vi "test SSL Client Read Before Write.vi"(8 "error in (no error)":errorcluster, 11 "TestCase in":refnum<class "test SSL Client.lvclass">) -> (0 "error out":errorcluster, 3 "TestCase out":refnum<class "test SSL Client.lvclass">)   [LabVIEW 2013, in "test SSL Client.lvclass"]
uses:
  test SSL Client.lvclass
  <vilib>/addons/_JKI Toolkits/VI Tester/TestCase.llb/TestCase.lvclass
  SSL_Lib/BIO/BIO.lvclass
  <vilib>/Utility/error.llb/DialogType.ctl
  SSL_Lib/SSL-Context/SSL-Context.lvclass
  SSL_Lib/SSL/SSL.lvclass
  SSL_Lib/SSL/SSL_Mode.ctl
  suite SSL Client/suite SSL Client/SSL Context.vi
  suite SSL Client/suite SSL Client/suite SSL Client.lvclass
  SSL_Lib/SSL-Lib/SSL-Lib.lvclass
panel:
  out "x-y":u32
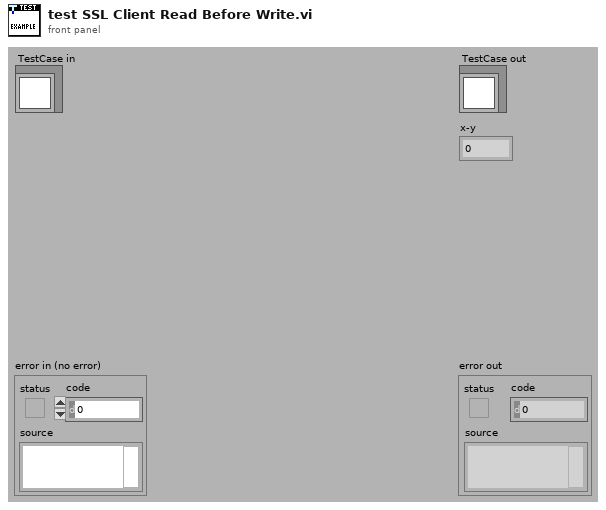
[diagram p1: front panel]
types:
  T1 = typedef "SSL_Lib.lvlib/SSL.lvclass/SSL_Mode.ctl" = i32
  T2 = typedef "DialogType.ctl" = u16
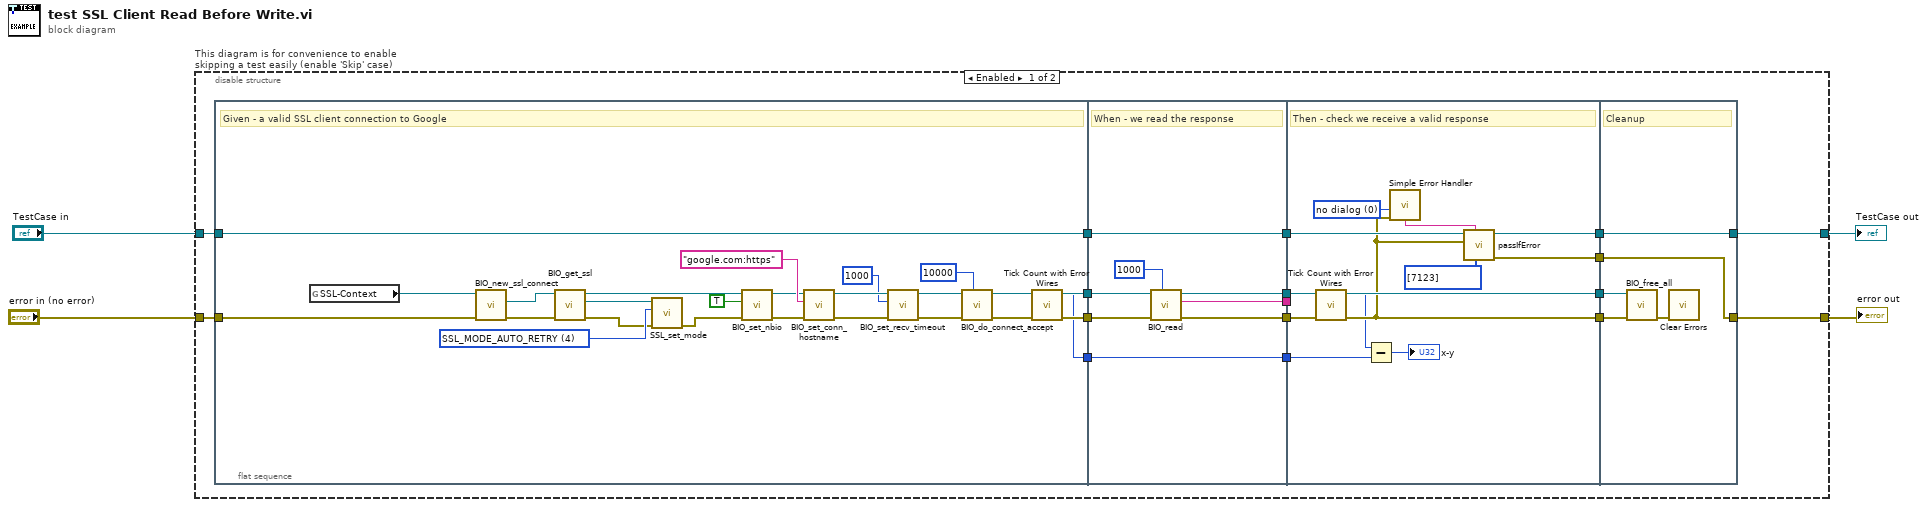
[diagram p0: block diagram]
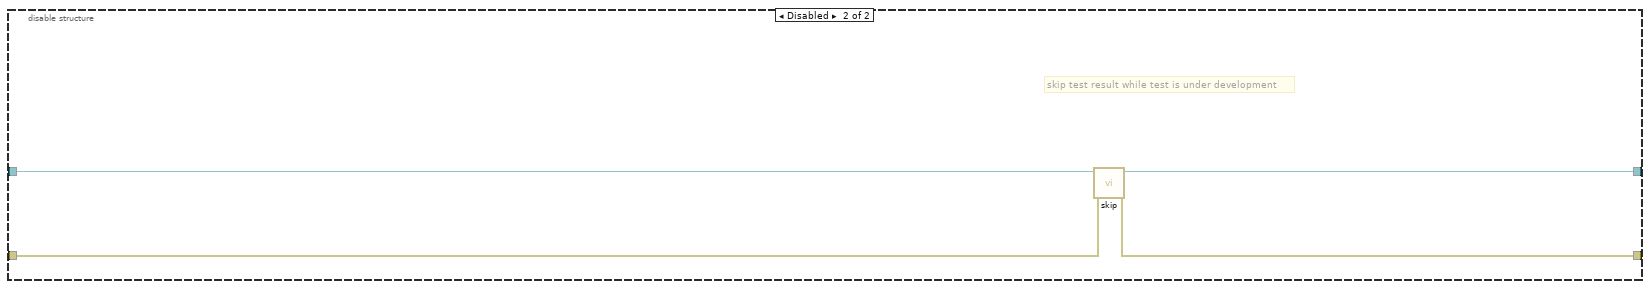
[diagram p2: hidden frame]
diagram:
  n1 = disable-structure "This diagram is for convenience to enable skipping a test easily (enable 'Skip' case)" shown="Enabled" {
    disable-tunnel: "TestCase in" -> [w16 w74]
    disable-tunnel: [w15 w72] -> w1
    disable-tunnel: [w14 w73] -> w3
    disable-tunnel: "error in (no error)" -> [w17 w71]
    frame Enabled {
      n2 = flat-sequence {
        tunnel: w17 -> [w37]
        tunnel: w16 -> [w36]
        tunnel: [w36] -> w21
        tunnel: [w28] -> w13
        tunnel: [w43] -> w12
        tunnel: [w27] -> w7
        tunnel: [w53] -> w20
        tunnel: [w50] -> w19
        tunnel: w21 -> [w53]
        tunnel: w13 -> [w52]
        tunnel: w12 -> [w51]
        tunnel: [w49] -> w11
        tunnel: [w48] -> w10
        tunnel: w7 -> [w46]
        tunnel: [w46] -> w6
        tunnel: [w64] -> w18
        tunnel: w20 -> [w65]
        tunnel: w19 -> [w60]
        tunnel: w11 -> [_]
        tunnel: w10 -> [w61]
        tunnel: [w61] -> w9
        tunnel: [w59] -> w8
        tunnel: w6 -> [w57]
        tunnel: [w54] -> w5
        tunnel: [w66] -> w14
        tunnel: [w70] -> w15
        tunnel: w18 -> [w70]
        tunnel: w9 -> [w68]
        tunnel: w8 -> [w69]
        tunnel: w5 -> [w66]
        frame #0 {
          w39 = T1 4 items=["None"=0, "SSL_MODE_ENABLE_PARTIAL_WRITE"=1, "SSL_MODE_ACCEPT_MOVING_WRITE_BUFFER"=2, "SSL_MODE_AUTO_RETRY"=4, "SSL_MODE_RELEASE_BUFFERS"=16, "SSL_MODE_SEND_FALLBACK_SCSV"=128] ("Mode")
          # "Given - a valid SSL client connection to Google"
          n3 = global read "SSL Context.vi" "SSL-Context"() -> (w35:refnum<class "SSL-Context.lvclass">)
          n4 = call "BIO_new_ssl_connect.vi"("error in (no error)"=w37, "SSL-Context in"=w35) -> ("error out"=w41:errorcluster, "BIO out"=w42:refnum<class "BIO.lvclass">)  [unwired: 7 in, 1 out]
          n5 = call "BIO_get_ssl.vi"("error in (no error)"=w41, "BIO in"=w42) -> ("error out"=w38:errorcluster, "SSL out"=w40:refnum<class "SSL.lvclass">, "BIO out"=w26:refnum<class "BIO.lvclass">)  [unwired: 7 in]
          n6 = call "SSL_set_mode.vi"("error in (no error)"=w38, "Mode"=w39, "SSL in"=w40) -> ("error out"=w24:errorcluster)  [unwired: 7 in, 1 out]
          n7 = call "BIO_set_nbio.vi"("error in (no error)"=w24, "Non-Blocking?"=TRUE, "BIO in"=w26) -> ("error out"=w23:errorcluster, "BIO out"=w25:refnum<class "BIO.lvclass">)  [unwired: 7 in]
          n8 = call "BIO_set_conn_hostname.vi"("error in (no error)"=w23, "Hostname"="google.com:https", "BIO in"=w25) -> ("error out"=w34:errorcluster, "BIO out"=w33:refnum<class "BIO.lvclass">)  [unwired: 7 in]
          n9 = call "BIO_set_recv_timeout.vi"("error in (no error)"=w34, "RECV timeout (ms)"=u32 1000, "BIO in"=w33) -> ("error out"=w31:errorcluster, "BIO out"=w32:refnum<class "BIO.lvclass">)  [unwired: 7 in]
          n10 = call "BIO_do_connect_accept.vi"("Timeout (10000ms)"=u32 10000, "error in (no error)"=w31, "BIO in"=w32) -> ("error out"=w29:errorcluster, "BIO out"=w43:refnum<class "BIO.lvclass">)  [unwired: 7 in]
          n11 = call "Tick Count with Error Wires.vi"("error in (no error)"=w29) -> ("error out"=w28:errorcluster, "millisecond timer value"=w27:u32)  [unwired: 9 in]
        }
        frame #1 {
          # "When - we read the response"
          n12 = call "BIO_read.vi"("Timeout (10000ms)"=u32 1000, "error in (no error)"=w52, "BIO in"=w51) -> ("error out"=w50:errorcluster, "String read"=w49:string, "BIO out"=w48:refnum<class "BIO.lvclass">)  [unwired: 6 in]
        }
        frame #2 {
          w62 = T2 0 items=["no dialog", "OK message", "continue or stop message", "OK message + warnings", "continue/stop + warnings"] ("type of dialog (OK msg:1)")
          # "Then - check we receive a valid response"
          n13 = call "Tick Count with Error Wires.vi"("error in (no error)"=w60) -> ("error out"=w59:errorcluster, "millisecond timer value"=w58:u32)  [unwired: 9 in]
          n14 = Subtract(x=w58, y=w57) -> (x-y=→"x-y":u32)
          n15 = call <vilib>:"Simple Error Handler.vi"("type of dialog (OK msg:1)"=w62, "error in (no error)"=w59) -> ("message"=w63:string)  [unwired: 3 in, 4 out]
          n16 = call-dynamic "passIfError.vi"("passing error codes (default = any error code)"=i32[] [7123], "custom report message (\"\")"=w63, "error"=w59, "TestCase in"=w65) -> ("error out"=w54:errorcluster, "TestCase out"=w64:refnum<class "test SSL Client.lvclass">)  [unwired: 6 in]
        }
        frame #3 {
          # "Cleanup"
          n17 = call "BIO_free_all.vi"("error in (no error)"=w69, "BIO in"=w68) -> ("error out"=w67:errorcluster)  [unwired: 9 in]
          n18 = call <vilib>:"Clear Errors.vi"("error in (no error)"=w67) -> ()  [unwired: 5 in, 2 out]
        }
      }
    }
    frame Disabled {
      # "skip test result while test is under development"
      n19 = call <vilib>:"skip.vi"("error in (no error)"=w71, "TestCase in"=w74) -> ("error out"=w73:errorcluster, "TestCase out"=w72:refnum<class "test SSL Client.lvclass">)  [unwired: 8 in]
    }
  }
  "error out" <- w3
  "TestCase out" <- w1
